vi "Home Filter Wheel.vi"(8 "error in (no error)":errorcluster, 10 "Motor":i32, 11 "Filter Wheel in":refnum<class "Filter Wheel.lvclass">) -> (0 "error out":errorcluster, 1 "Success":bool, 2 "Log":string, 3 "Filter Wheel out":refnum<class "Filter Wheel.lvclass">)   [LabVIEW 2024, in "Filter Wheel.lvclass"]
uses:
  Filter Wheel.lvclass
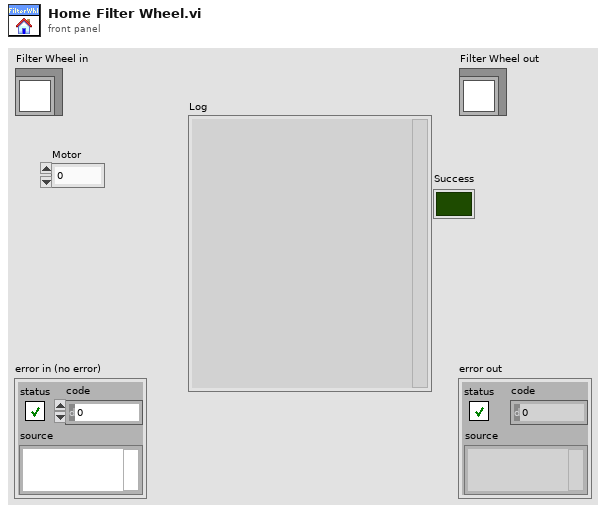
[diagram p1: front panel]
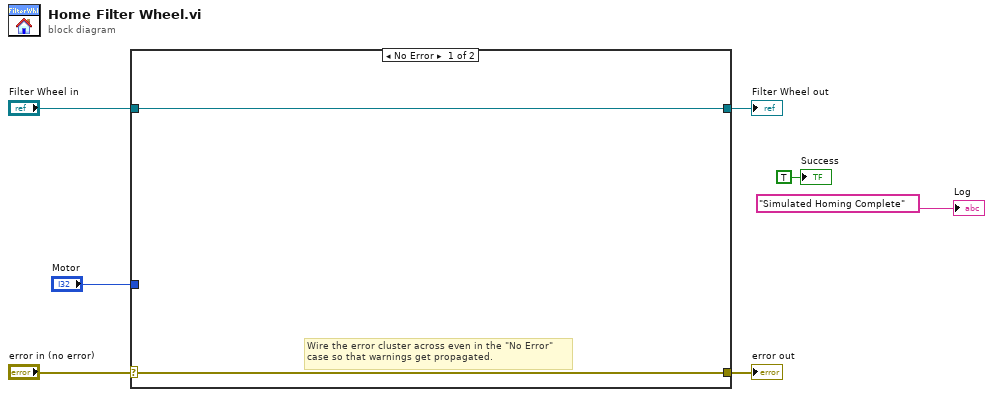
[diagram p0: block diagram]
diagram:
  n1 = case shown="No Error" "error in (no error)" {
    selector: "error in (no error)" -> [w9 w11]
    tunnel: [w9 w11] -> w6
    tunnel: [w8 w10] -> w4
    tunnel: "Filter Wheel in" -> [w8 w10]
    tunnel: "Motor" -> [_ _]
    frame No Error {
      # "Wire the error cluster across even in the \"No Error\"\ncase so that warnings get propagated."
    }
    frame Error {
    }
  }
  "error out" <- w6
  "Filter Wheel out" <- w4
  "Log" <- "Simulated Homing Complete"
  "Success" <- TRUE ("Success")
